vi "LV SciSDK FFT.vi"(8 "error in (no error)":errorcluster, 9 "FFT Handle In":T1) -> (0 "error out":errorcluster, 1 "FFT Handle Out":T1, 2 "buffer out":T2)   [LabVIEW 2021]
uses:
  SciSDK_Labview.lvlib
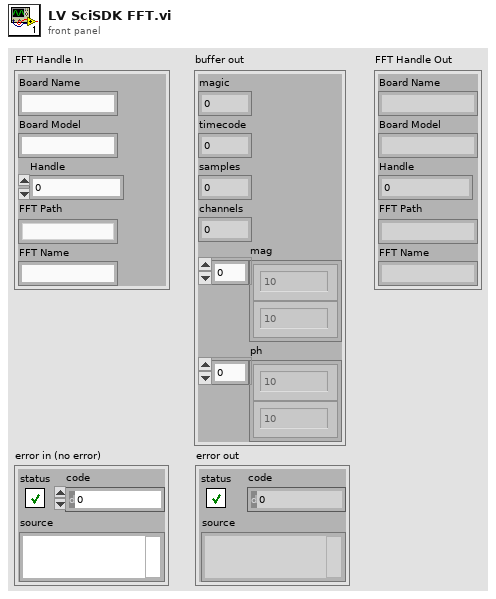
[diagram p1: front panel]
types:
  T1 = cluster{"Board Name":string, "Board Model":string, "Handle":u64, "FFT Path":string, "FFT Name":string}
  T2 = cluster{"magic":u32, "timecode":u32, "samples":u32, "channels":u32, "mag":dbl[], "ph":dbl[]}
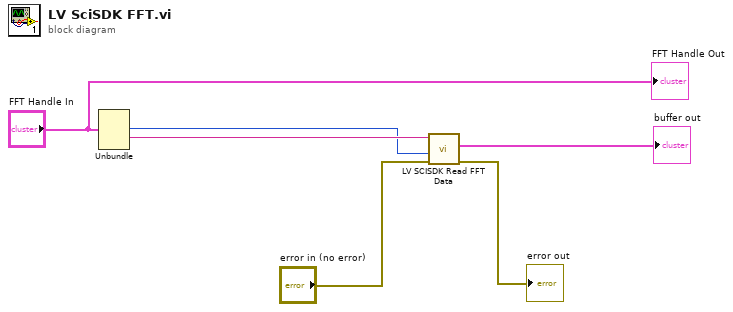
[diagram p0: block diagram]
diagram:
  n1 = Unbundle("FFT Handle In") -> ("Handle"=w5:u64, "FFT Path"=w6:string)  [unwired: 3 out]
  n2 = call "LV SCISDK Read FFT Data.vi"("Path"=w6, "handle"=w5, "error in (no error)"="error in (no error)") -> ("buffer out"=→"buffer out":T2, "error out"=→"error out":errorcluster)  [unwired: 4 in, 2 out]
  "FFT Handle Out" <- "FFT Handle In"
